vi "Detect Hardware.vi"(8 "error in (no error)":errorcluster, 11 "Microscope_RM21 in":refnum<class "Microscope_RM21.lvclass">) -> (0 "error out":errorcluster, 3 "Microscope_RM21 out":refnum<class "Microscope_RM21.lvclass">)   [LabVIEW 2020, in "Microscope_RM21.lvlib" / "Microscope_RM21.lvclass"]
uses:
  Microscope_RM21.lvclass
  D:/Daguan/Development/MMicroscopyAF/Model/HAL Layer/Microscope/Microscope/Microscope.lvclass
  Stage_MadCityLab/Stage_MadCityLab/Stage_MadCityLab.lvclass
  D:/Daguan/Development/MMicroscopyAF/Model/HAL Layer/Component/Device/Device/Device.lvclass
  <vilib>/ActorFramework/Message Enqueuer/Message Enqueuer.lvclass/Message Enqueuer.ctl
  Stage_MadCityLabMicro/Stage_MadCityLabMicro/Stage_MadCityLabMicro.lvclass
  DAQ_QPT_Throlab/DAQ_QPT_Throlab/DAQ_QPT_Throlab.lvclass
  Camera_Prime95B/Camera_Prime95B/Camera_Prime95B.lvclass
  Laser_Oxxius/Laser_Oxxius/Laser_Oxxius.lvclass
  <vilib>/ActorFramework/Message Enqueuer/Enqueue.vi
  HAL Layer/Component/Stage/Stage Messages/Start Sequence Acquisition Msg/Start Sequence Acquisition Msg.lvclass
  C:/Program Files/National Instruments/LabVIEW 2020/vi.lib/ActorFramework/Message/Message.lvclass
  HAL Layer/Component/DAQ/DAQ Messages/Start Sequence Acquisition Msg/Start Sequence Acquisition Msg.lvclass
  <vilib>/ActorFramework/Message Priority Queue/Priority Enqueue.vi
  HAL Layer/Microscope/Microscope/Microscope.lvclass
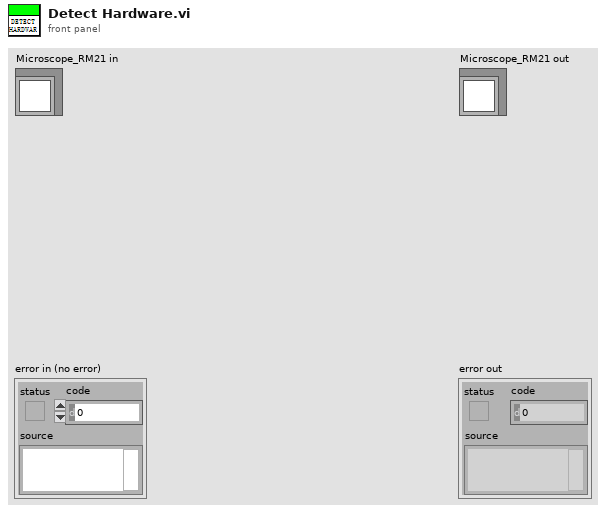
[diagram p1: front panel]
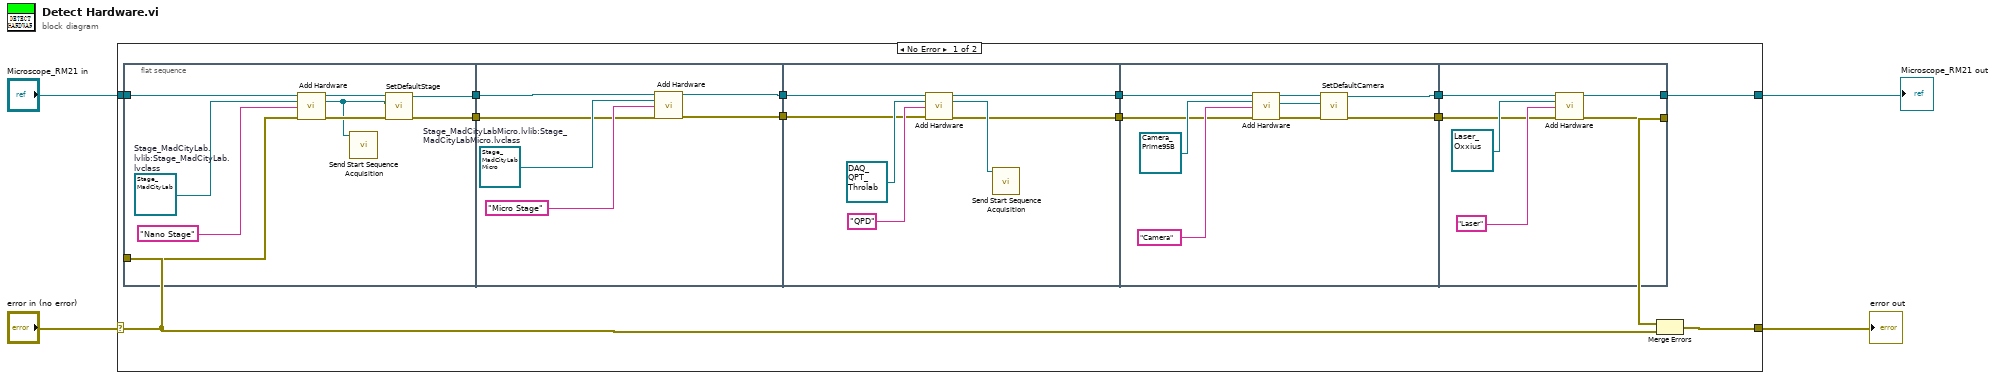
[diagram p0: block diagram]
diagram:
  n1 = case shown="No Error" "error in (no error)" {
    selector: "error in (no error)" -> [w13 w56]
    tunnel: [w14 w56] -> w3
    tunnel: "Microscope_RM21 in" -> [w17 w55]
    tunnel: [w15 w55] -> w1
    frame No Error {
      n2 = flat-sequence {
        tunnel: w17 -> [w26]
        tunnel: [w19] -> w16
        tunnel: w13 -> [w25]
        tunnel: [w21] -> w11
        tunnel: w16 -> [w32]
        tunnel: [w31] -> w12
        tunnel: w11 -> [w28]
        tunnel: [w27] -> w10
        tunnel: w12 -> [w38]
        tunnel: w10 -> [w35]
        tunnel: [w37] -> w9
        tunnel: [w33] -> w7
        tunnel: w9 -> [w48]
        tunnel: [w41] -> w8
        tunnel: w7 -> [w45]
        tunnel: [w43] -> w6
        tunnel: [w53] -> w15
        tunnel: w8 -> [w54]
        tunnel: w6 -> [w50]
        tunnel: [w49] -> w5
        frame #0 {
          w23 = refnum<class "Stage_MadCityLab.lvclass"> refnum  # Stage_MadCityLab.lvlib:Stage_MadCityLab.lvclass
          n3 = call "Add Hardware.vi"("Microscope in"=w26, "Device.lvlib:Device.lvclass"=w23, "Label"="Nano Stage" ("Sub Panel"), "error in (no error)"=w25) -> ("Microscope out"=w20:refnum<class "Microscope_RM21.lvclass">, "Nested Actor's Enqueuer"=w18:refnum<class "Message Enqueuer.lvclass">, "error out"=w22:errorcluster)  [unwired: 7 in, 2 out]
          n4 = call "Send Start Sequence Acquisition.vi"("Message Enqueuer"=w18) -> ()  [unwired: 9 in, 2 out]
          n5 = call-dynamic "SetDefaultStage.vi"("error in (no error)"=w22, "DefaultStageEnqueuer"=w18, "Microscope in"=w20) -> ("error out"=w21:errorcluster, "Microscope out"=w19:refnum<class "Microscope_RM21.lvclass">)  [unwired: 7 in]
        }
        frame #1 {
          w30 = refnum<class "Stage_MadCityLabMicro.lvclass"> refnum  # Stage_MadCityLabMicro.lvlib:Stage_MadCityLabMicro.lvclass
          n6 = call "Add Hardware.vi"("Microscope in"=w32, "Device.lvlib:Device.lvclass"=w30, "Label"="Micro Stage" ("Sub Panel"), "error in (no error)"=w28) -> ("Microscope out"=w31:refnum<class "Microscope_RM21.lvclass">, "error out"=w27:errorcluster)  [unwired: 7 in, 3 out]
        }
        frame #2 {
          n7 = call "Add Hardware.vi"("Microscope in"=w38, "Device.lvlib:Device.lvclass"=refnum<class "DAQ_QPT_Throlab.lvclass"> refnum ("DAQ_QPT_Throlab.lvlib:DAQ_QPT_Throlab.lvclass"), "Label"="QPD", "error in (no error)"=w35) -> ("Microscope out"=w37:refnum<class "Microscope_RM21.lvclass">, "Nested Actor's Enqueuer"=w34:refnum<class "Message Enqueuer.lvclass">, "error out"=w33:errorcluster)  [unwired: 7 in, 2 out]
          n8 = call "Send Start Sequence Acquisition.vi"("Message Enqueuer"=w34) -> ()  [unwired: 9 in, 2 out]
        }
        frame #3 {
          n9 = call "Add Hardware.vi"("Microscope in"=w48, "Device.lvlib:Device.lvclass"=refnum<class "Camera_Prime95B.lvclass"> refnum ("Camera_Prime95B.lvlib:Camera_Prime95B.lvclass"), "Label"="Camera", "error in (no error)"=w45) -> ("Microscope out"=w42:refnum<class "Microscope_RM21.lvclass">, "Nested Actor's Enqueuer"=w40:refnum<class "Message Enqueuer.lvclass">, "error out"=w44:errorcluster)  [unwired: 7 in, 2 out]
          n10 = call-dynamic "SetDefaultCamera.vi"("error in (no error)"=w44, "DefaultCameraEnqueuer"=w40, "Microscope in"=w42) -> ("error out"=w43:errorcluster, "Microscope out"=w41:refnum<class "Microscope_RM21.lvclass">)  [unwired: 7 in]
        }
        frame #4 {
          n11 = call "Add Hardware.vi"("Microscope in"=w54, "Device.lvlib:Device.lvclass"=refnum<class "Laser_Oxxius.lvclass"> refnum ("Laser_Oxxius.lvlib:Laser_Oxxius.lvclass"), "Label"="Laser", "error in (no error)"=w50) -> ("Microscope out"=w53:refnum<class "Microscope_RM21.lvclass">, "error out"=w49:errorcluster)  [unwired: 7 in, 3 out]
        }
      }
      n12 = Merge Errors(w5, w13) -> (w14:errorcluster)
    }
    frame Error {
    }
  }
  "error out" <- w3
  "Microscope_RM21 out" <- w1
